vi "Menu.Help, Open User Manual Items.vi"(8 "error in (no error)":errorcluster, 9 "Menu Tag Selection":string, 10 "Paths":path[](array[path]), 11 "Tags":string[](array[string])) -> (0 "error out":errorcluster)   [LabVIEW 2024, in "EQMF.lvlib" / "Menu Utils.lvlib"]
uses:
  Menu Utils.lvlib
  Files/File Utils.lvlib
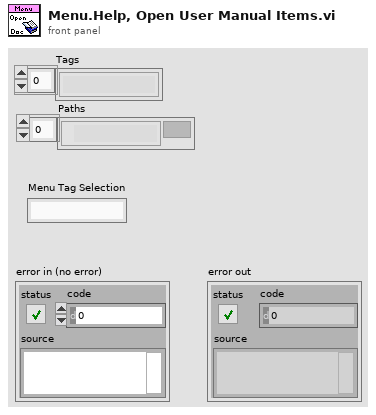
[diagram p1: front panel]
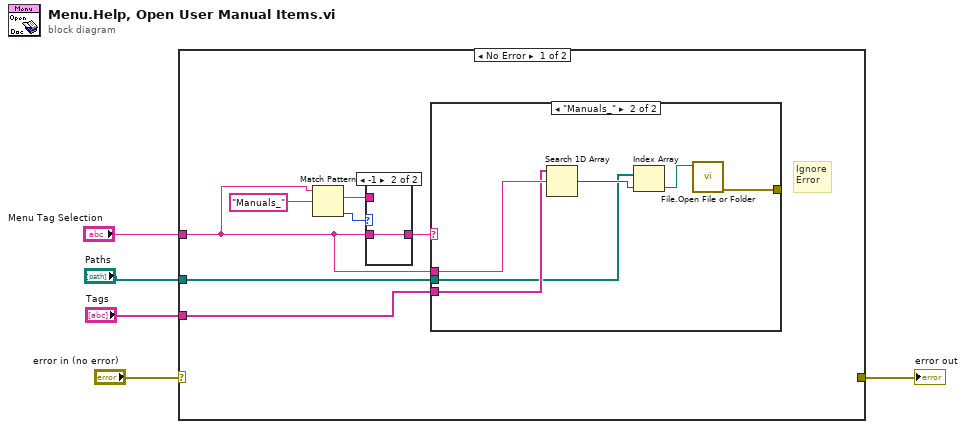
[diagram p0: block diagram]
diagram:
  n1 = case shown="No Error" "error in (no error)" {
    selector: "error in (no error)" -> [_ w21]
    tunnel: "Paths" -> [w8 _]
    tunnel: "Tags" -> [w7 _]
    tunnel: "Menu Tag Selection" -> [w6 _]
    tunnel: [_ w21] -> w1
    frame No Error {
      # "Ignore\nError"
      n2 = Match Pattern(string=w6, regular expression="Manuals_") -> (match substring=w12:string, offset past match=w11:i32)  [unwired: 1 in, 2 out]
      n3 = case shown="-1" w11 {
        tunnel: w6 -> [_ w20]
        tunnel: [w19 w20] -> w9
        tunnel: w12 -> [w19 _]
        frame 0, Default {
        }
        frame -1 {
        }
      }
      n4 = case shown="\"Manuals_\"" w9 {
        tunnel: w7 -> [_ w15]
        tunnel: w6 -> [_ w16]
        tunnel: w8 -> [_ w14]
        tunnel: [_ w13] -> _
        frame Default {
          # "Do Nothing"
        }
        frame "Manuals_" {
          n5 = Search 1D Array(1D array=w15, element=w16) -> (index of element=w17:i32)  [unwired: 1 in]
          n6 = Index Array(array=w14, index=w17) -> (element=w18:path)
          n7 = call "File.Open File or Folder.vi"("Path"=w18) -> ("Error Out"=w13:errorcluster)  [unwired: 10 in]
        }
      }
    }
    frame Error {
    }
  }
  "error out" <- w1
